vi "Start Stream.vi"(8 "Error In":errorcluster) -> (0 "Error Out":errorcluster, 3 "Command":u8[](array[numeric]) format="%02x")   [LabVIEW 2012]
uses:
  Controls/Desciptor Set Byte.ctl
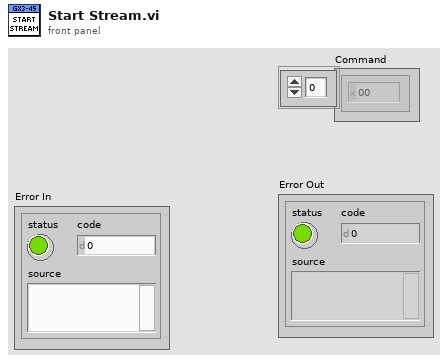
[diagram p1: front panel]
types:
  T1 = typedef "Desciptor Set Byte.ctl" = enum16{"Base Command Set", "3DM Command Set", "Navigation Filter Command Set", "System Command Set", "AHRS", "GPS", "NAV"}
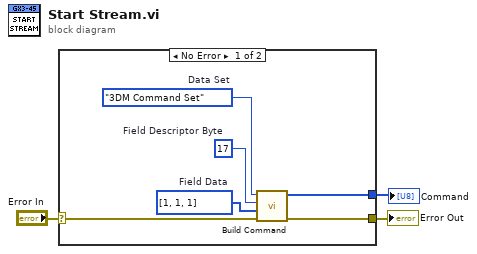
[diagram p0: block diagram]
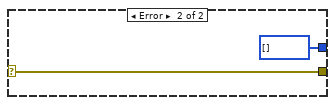
[diagram p2: hidden frame]
diagram:
  n1 = case shown="No Error" "Error In" {
    selector: "Error In" -> [w6 w11]
    tunnel: [w5 w11] -> w2
    tunnel: [w4 u8[] [] ("Command")] -> w1
    frame No Error {
      w7 = u8[] [1, 1, 1]  # Field Data
      w8 = u8 17  # Field Descriptor Byte
      w9 = Desciptor_Set_Byte."3DM Command Set"  # Data Set
      n2 = call "Build Command.vi"("Error In"=w6, "Field Data"=w7, "Field Descriptor Byte"=w8, "Data Set"=w9) -> ("Error Out"=w5:errorcluster, "Command"=w4:u8[])  [unwired: 6 in]
    }
    frame Error {
    }
  }
  "Error Out" <- w2
  "Command" <- w1
